vi "LVPortIncludeLibPaths.vi"(8 "error in (no error)":errorcluster, 10 "Include Paths":path[](array[path]), 11 "Include path":path) -> (0 "error out":errorcluster)   [LabVIEW 2017]
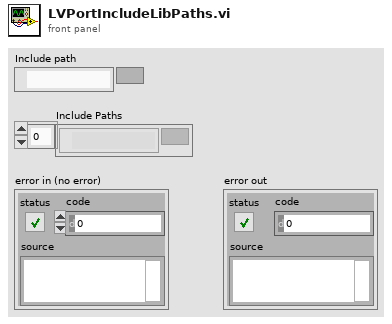
[diagram p1: front panel]
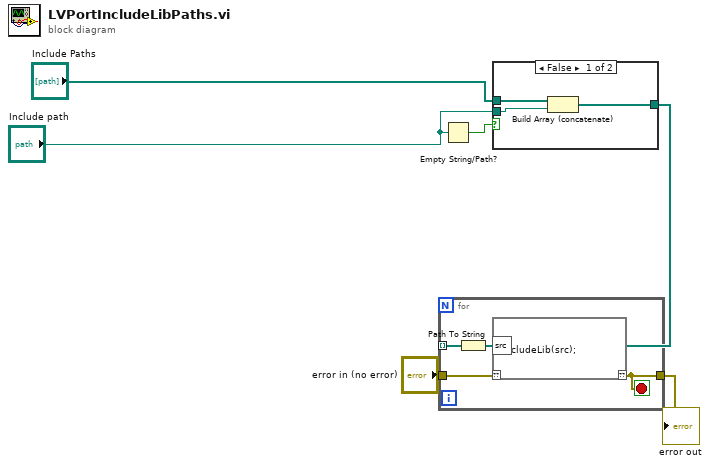
[diagram p0: block diagram]
diagram:
  n1 = Empty String/Path?(string/path="Include path") -> (empty?=w1:bool)
  n2 = case shown="False" w1 {
    tunnel: "Include Paths" -> [w9 w10]
    tunnel: "Include path" -> [w8 _]
    tunnel: [w7 w10] -> w4
    frame False {
      n3 = Build Array (concatenate)(w9, w8) -> (w7:path[])
    }
    frame True {
    }
  }
  n4 = for {
    tunnel: w4 -> [w14] mode=indexing
    tunnel: "error in (no error)" -> [w12]
    tunnel: [w11] -> w6
    stop <- w11 stop-if-true
    n5 = Path To String(path=w14) -> (string=w13:string)
    n6 = script code="IncludeLib(src);"("??"=w12, "src"=w13) -> ("??"=w11:errorcluster)
  }
  "error out" <- w6
